vi "midi_winapi_idtech1.vi"(9 "stop":bool, 10 "Beat(Hz)":i32) -> (0 "error out":errorcluster, 2 "MIDI output handle":i32)   [LabVIEW 8.6]
uses:
  winmm.dll
panel:
  out "Event":u8 format="%.0x"
  out "Note":u8
  out "Vol":u8
  out "Channel":u8
  out "count":i32
  out "Graph":u8[][](graph)
  in  "error in":errorcluster
  in  "Maps":enum16{"E1M1", "E1M2", "E1M3", "E1M9"}(ring)
  out "Events":i32
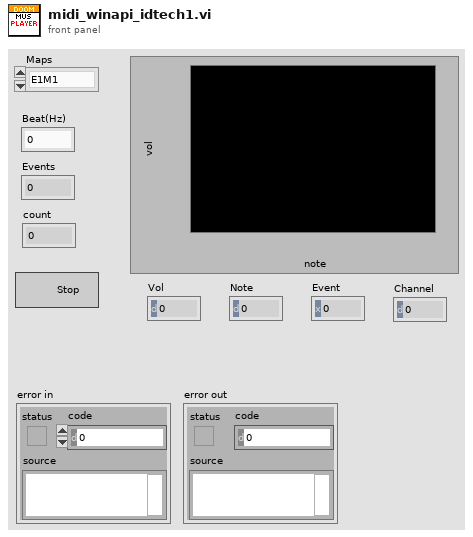
[diagram p1: front panel]
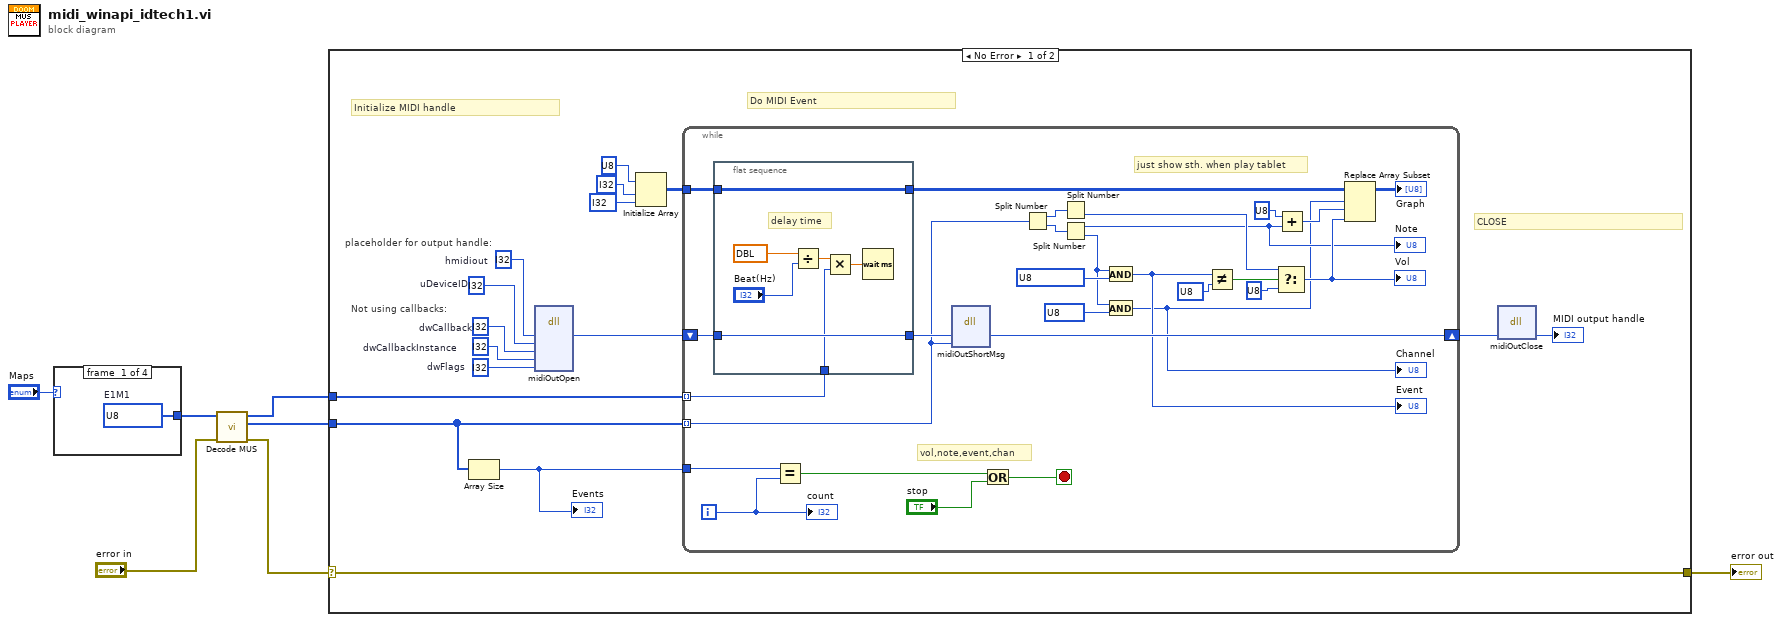
[diagram p0: block diagram]
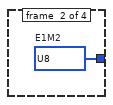
[diagram p2: hidden frame]
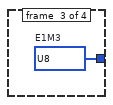
[diagram p3: hidden frame]
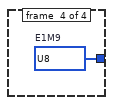
[diagram p4: hidden frame]
diagram:
  n1 = case shown="\"E1M2\"" "Maps" {
    tunnel: [w8 w9 w10 w11] -> w2
    frame #0 {
      w8 = u8[] ?  # E1M1
    }
    frame #1 {
      w9 = u8[] ?  # E1M2
    }
    frame #2 {
      w10 = u8[] ?  # E1M3
    }
    frame #3 {
      w11 = u8[] ?  # E1M9
    }
  }
  n2 = call "Decode MUS.vi"("error in"="error in", "Music_Lump in"=w2) -> ("error out"=w5:errorcluster, "midi_Msg"=w6:u32[], "delay"=w7:u32[])  [unwired: 7 in]
  n3 = case shown="No Error" w5 {
    selector: w5 -> [w16 w63]
    tunnel: w7 -> [w19 _]
    tunnel: w6 -> [w18 _]
    tunnel: [w16 w63] -> w4
    frame #0 {
      w26 = i32 ?  # uDeviceID
      w23 = i32 ?  # dwFlags
      w24 = i32 ?  # dwCallbackInstance
      w25 = i32 ?  # dwCallback
      w27 = i32 ?  # hmidiout
      # "Initialize MIDI handle"
      # "Do MIDI Event"
      # "CLOSE"
      # "placeholder for output handle:"
      # "Not using callbacks:"
      n4 = Array Size(array=w18) -> (size(s)=w17:i32)
      "Events" <- w17
      n5 = dll-call lib="winmm.dll" fn="midiOutOpen"("hmidiout"=w27, "uDeviceID"=w26, "dwCallback"=w25, "dwCallbackInstance"=w24, "dwFlags"=w23) -> ("hmidiout"=w20:i32)  [unwired: 8 in, 2 out]
      n6 = Initialize Array(u8 ?, i32 ? ("index"), i32 ? ("index")) -> (w12:u8[][])
      n7 = while {
        shift-right: [w55] -> w21
        shift-left: w20 -> [w54]
        tunnel: w19 -> [w51] mode=indexing
        tunnel: w18 -> [w46] mode=indexing
        tunnel: w17 -> [w50]
        tunnel: w12 -> [w47]
        i -> [w33]
        stop <- w52 stop-if-true
        # "just show sth. when play tablet"
        # "vol,note,event,chan"
        n8 = flat-sequence {
          tunnel: w54 -> [w62]
          tunnel: [w62] -> w53
          tunnel: w51 -> [w57]
          tunnel: w47 -> [w56]
          tunnel: [w56] -> w38
          frame #0 {
            # "delay time"
            n9 = Divide(x=dbl ?, y="Beat(Hz)") -> (x/y=w61:dbl)
            n10 = Multiply(x=w61, y=w57) -> (x*y=w58:dbl)
            n11 = Wait (ms)(milliseconds to wait=w58) -> ()  [unwired: 1 out]
          }
        }
        n12 = Equal?(x=w50, y=w33) -> (x = y?=w49:bool)
        n13 = dll-call lib="winmm.dll" fn="midiOutShortMsg"("hmidiout"=w53, "data"=w46) -> ("hmidiout"=w55:i32)  [unwired: 5 in, 2 out]
        n14 = Or(x=w49, y="stop") -> (x .or. y?=w52:bool)
        n15 = Split Number(x=w46) -> (hi(x)=w45:u16, lo(x)=w44:u16)
        n16 = Split Number(x=w45) -> (lo(x)=w37:u8)  [unwired: 1 out]
        n17 = Split Number(x=w44) -> (hi(x)=w29:u8, lo(x)=w41:u8)
        "Note" <- w29
        n18 = And(x=w41, y=u8 ? ("f")) -> (x .and. y?=w30:u8)
        "Event" <- w30
        n19 = And(x=w41, y=u8 ? ("f")) -> (x .and. y?=w28:u8)
        "Channel" <- w28
        n20 = Not Equal?(x=w30, y=u8 ?) -> (x != y?=w40:bool)
        n21 = Select(t=w37, s=w40, f=u8 ?) -> (s? t:f=w36:u8)
        "Vol" <- w36
        n22 = Add(x=u8 ?, y=w29) -> (x+y=w34:u8)
        n23 = Replace Array Subset(array=w38, new element=w36, index (row)=w28, index (col)=w34) -> (→"Graph":u8[][])
        "count" <- w33
      }
      n24 = dll-call lib="winmm.dll" fn="midiOutClose"("hmidiout"=w21) -> ("hmidiout"=→"MIDI output handle":i32)  [unwired: 4 in, 2 out]
    }
    frame #1 {
    }
  }
  "error out" <- w4
